vi "生成任务队列.vi"(10 "循环次数":u32, 11 "循环等待":u32=500) -> (2 "任务数据":variant[](array[variant]), 3 "任务名称":string[](array[string]))   [LabVIEW 2020]
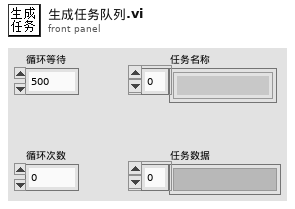
[diagram p1: front panel]
types:
  T1 = enum8{"Enabled", "Disabled", "Disabled and Grayed Out"}
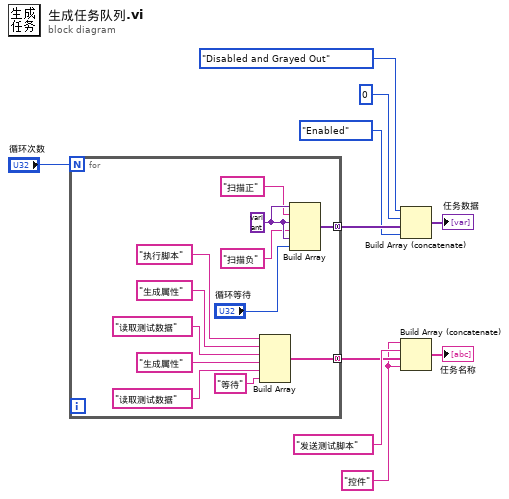
[diagram p0: block diagram]
diagram:
  w2 = "控件" ("元素")
  n1 = for {
    N: "循环次数" -> [_]
    tunnel: [w13] -> w8 mode=concatenating
    tunnel: [w12] -> w5 mode=concatenating
    w16 = variant ("元素")
    n2 = Build Array("执行脚本" ("消息"), "生成属性" ("消息"), "读取测试数据" ("消息"), "生成属性" ("消息"), "读取测试数据" ("消息"), "等待" ("元素")) -> (w13:string[])
    n3 = Build Array(w16, "扫描正" ("消息"), w16, "扫描负" ("消息"), w16, "循环等待") -> (w12:variant[])
  }
  n4 = Build Array (concatenate)(T1."Disabled and Grayed Out" ("禁用"), 0, w5, T1."Enabled" ("禁用")) -> (→"任务数据":variant[])
  n5 = Build Array (concatenate)(w2, "发送测试脚本" ("消息"), w8, w2) -> (→"任务名称":string[])
